vi "SetGraphTime.vi"(8 "error in (no error)":errorcluster, 11 "Gviewer in":refnum<class "Gviewer.lvclass">) -> (0 "error out":errorcluster, 3 "Gviewer out":refnum<class "Gviewer.lvclass">)   [LabVIEW 2020, in "Sgraph_lib_V1.lvlib" / "Gviewer.lvclass"]
doc: "Set XY graph X scale (time) left and right"
uses:
  Gviewer.lvclass
  Gviewer.lvclass/Gviewer.ctl
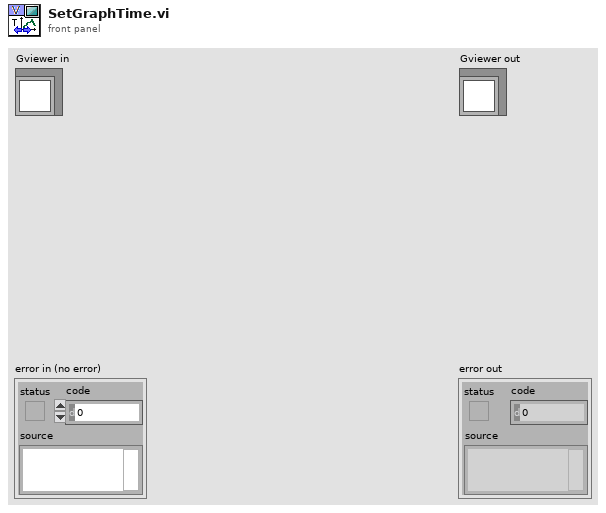
[diagram p1: front panel]
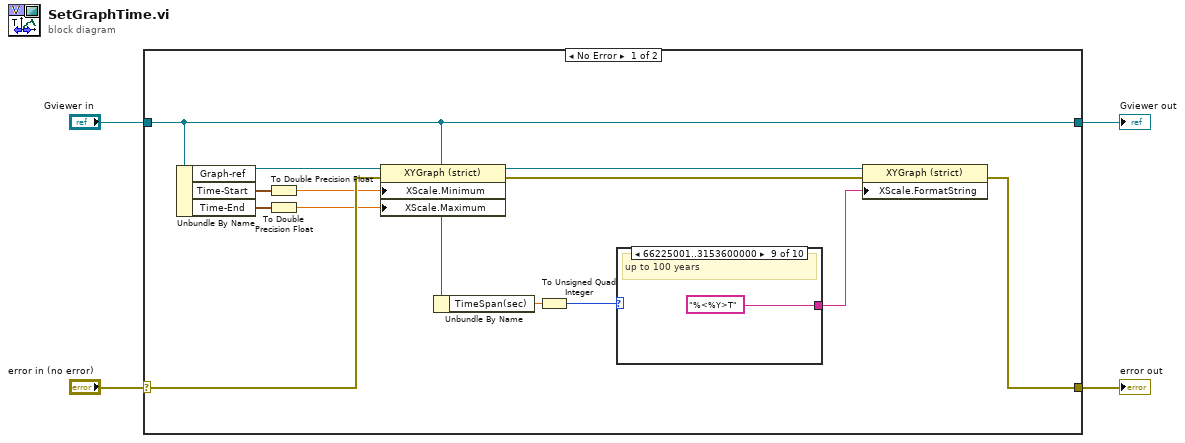
[diagram p0: block diagram]
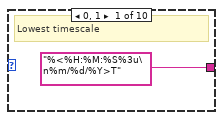
[diagram p2: hidden frame]
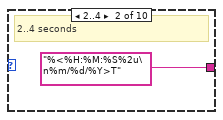
[diagram p3: hidden frame]
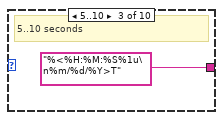
[diagram p4: hidden frame]
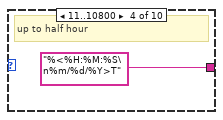
[diagram p5: hidden frame]
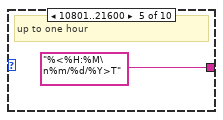
[diagram p6: hidden frame]
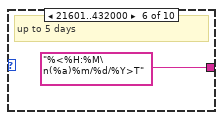
[diagram p7: hidden frame]
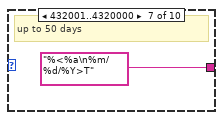
[diagram p8: hidden frame]
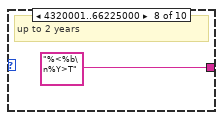
[diagram p9: hidden frame]
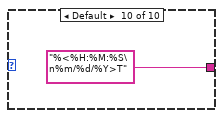
[diagram p10: hidden frame]
diagram:
  n1 = case shown="No Error" "error in (no error)" {
    selector: "error in (no error)" -> [w16 w29]
    tunnel: [w15 w29] -> w3
    tunnel: [w17 w28] -> w1
    tunnel: "Gviewer in" -> [w17 w28]
    frame No Error {
      n2 = Unbundle By Name(w17) -> ("Graph-ref"=w11:refnum<vi>, "Time-Start"=w7:timestamp, "Time-End"=w8:timestamp)
      n3 = To Double Precision Float(number=w7) -> (double precision float=w6:dbl)
      n4 = To Double Precision Float(number=w8) -> (double precision float=w5:dbl)
      n5 = property class="XYGraph (strict)"(reference=w11, error in=w16, "XScale.Minimum"=w6, "XScale.Maximum"=w5) -> (reference out=w9:refnum<vi>, error out=w10:errorcluster)
      n6 = Unbundle By Name(w17) -> ("TimeSpan(sec)"=w12:dbl)
      n7 = To Unsigned Quad Integer(1:w12) -> (0:w13:u64)
      n8 = case shown="66225001..3153600000" w13 {
        tunnel: ["%<%H:%M:%S%3u\n%m/%d/%Y>T" "%<%H:%M:%S%2u\n%m/%d/%Y>T" "%<%H:%M:%S%1u\n%m/%d/%Y>T" "%<%H:%M:%S\n%m/%d/%Y>T" "%<%H:%M\n%m/%d/%Y>T" "%<%H:%M\n(%a)%m/%d/%Y>T" "%<%a\n%m/%d/%Y>T" "%<%b\n%Y>T" "%<%Y>T" "%<%H:%M:%S\n%m/%d/%Y>T"] -> w14
        frame 0, 1 {
          # "Lowest timescale"
        }
        frame 2..4 {
          # "2..4 seconds"
        }
        frame 5..10 {
          # "5..10 seconds"
        }
        frame 11..10800 {
          # "up to half hour"
        }
        frame 10801..21600 {
          # "up to one hour"
        }
        frame 21601..432000 {
          # "up to 5 days"
        }
        frame 432001..4320000 {
          # "up to 50 days"
        }
        frame 4320001..66225000 {
          # "up to 2 years"
        }
        frame 66225001..3153600000 {
          # "up to 100 years"
        }
        frame Default {
        }
      }
      n9 = property class="XYGraph (strict)"(reference=w9, error in=w10, "XScale.FormatString"=w14) -> (error out=w15:errorcluster)  [unwired: 1 out]
    }
    frame Error {
    }
  }
  "error out" <- w3
  "Gviewer out" <- w1
